vi "Analysis Info Cluster from String.vi"(7 "Setup String":string) -> (0 "Initial Probe Positions":T8[](array[typedef]), 1 "Dynamically Added":T1[](array[typedef]) {"Fs" format="%#_pHz"; "syncDelay" format="%#_gms"; "Ch" min=0 step=1}, 2 "XYZ Positions":dbl[][](array[numeric]), 3 "Ch & spans choices":T1[](array[typedef]) {"Fs" format="%#_pHz"; "syncDelay" format="%#_gms"; "Ch" min=0 step=1}, 4 "Initial Info Cluster":T7[](array[typedef]), 5 "Number of Analogue instruments":i32=1, 6 "Acquisition_Plugin":string[](array[string]), 8 "LDA Setup":T1[](array[typedef]) {"Fs" format="%#_pHz"; "syncDelay" format="%#_gms"; "Ch" min=0 step=1})   [LabVIEW 2022 SP3]
uses:
  Controls/Meas input Cluster.ctl
  Controls/Inst_type.ctl
  Controls/portOrDev.ctl
  Controls/calType.ctl
  Controls/channelState.ctl
  Controls/DAQinputType.ctl
  Controls/Initial Positions.ctl
  Controls/Initial Info Cluster.ctl
  Globals/Meas_global.vi
panel:
  in  "Inst type":T2=enum."Propeller anemometer"
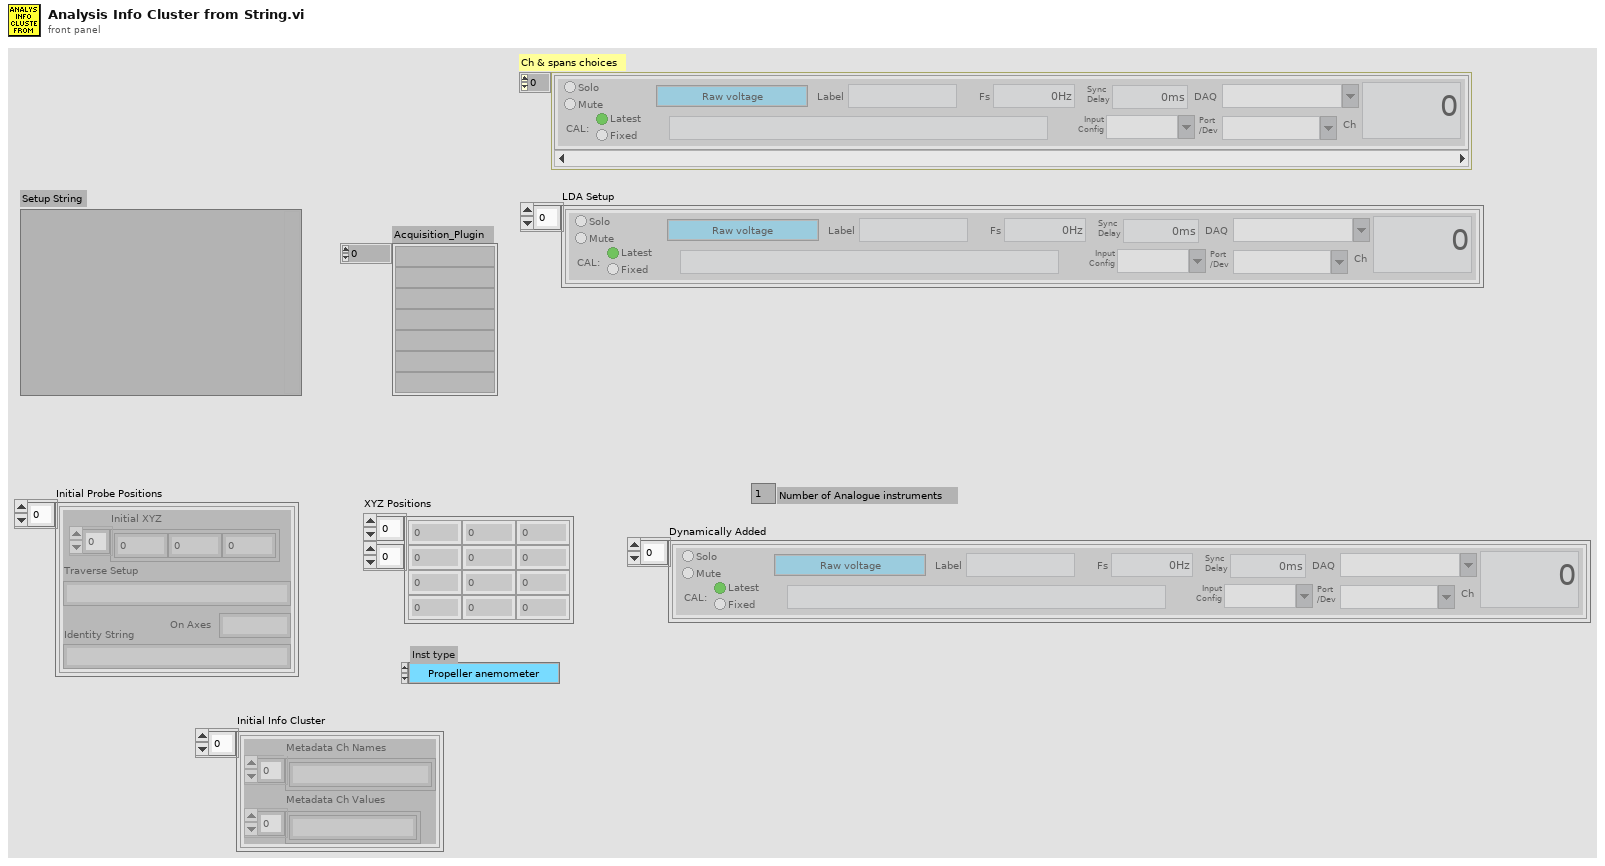
[diagram p1: front panel]
types:
  T1 = typedef "Meas input Cluster.ctl" = cluster{"Type":T2, "Label":string, "DAQ":string, "Port":T3, "Ch":i32, "Cal":path, "calType":T4, "Fs":dbl, "syncDelay":dbl, "chState":T5, "inputConfig":T6}
  T2 = typedef "Inst_type.ctl" = enum16{"Raw voltage", "Raw with zero offsetting", "Propeller anemometer", "Pressure Transducer", "Pitot-static tube", "Hot wire", "Cross wire 1", "Cross wire 2", "Generic Linear", "Generic Polynomial", "Generic BackPoly", "Fast FID", "Thermocouple", "Cold wire", "Pulsed Wire", "LDA Vel", "LDA Tran time", "LDA Arr time", "Microphone"}
  T3 = typedef "portOrDev.ctl" = string
  T4 = typedef "calType.ctl" = enum32{"Latest", "Fixed"}
  T5 = typedef "channelState.ctl" = enum32{"No Selection", "Solo", "Mute"}
  T6 = typedef "DAQinputType.ctl" = string
  T7 = typedef "Initial Info Cluster.ctl" = cluster{"Metadata Ch Names":string[], "Metadata Ch Values":string[]}
  T8 = typedef "Initial Positions.ctl" = cluster{"Initial XYZ":sgl[], "Traverse Setup":string, "On Axes":string, "Identity String":string}
  T9 = typedef "Post_Process.ctl" = enum16{"Take New Data", "Post Process Raw Data File"}
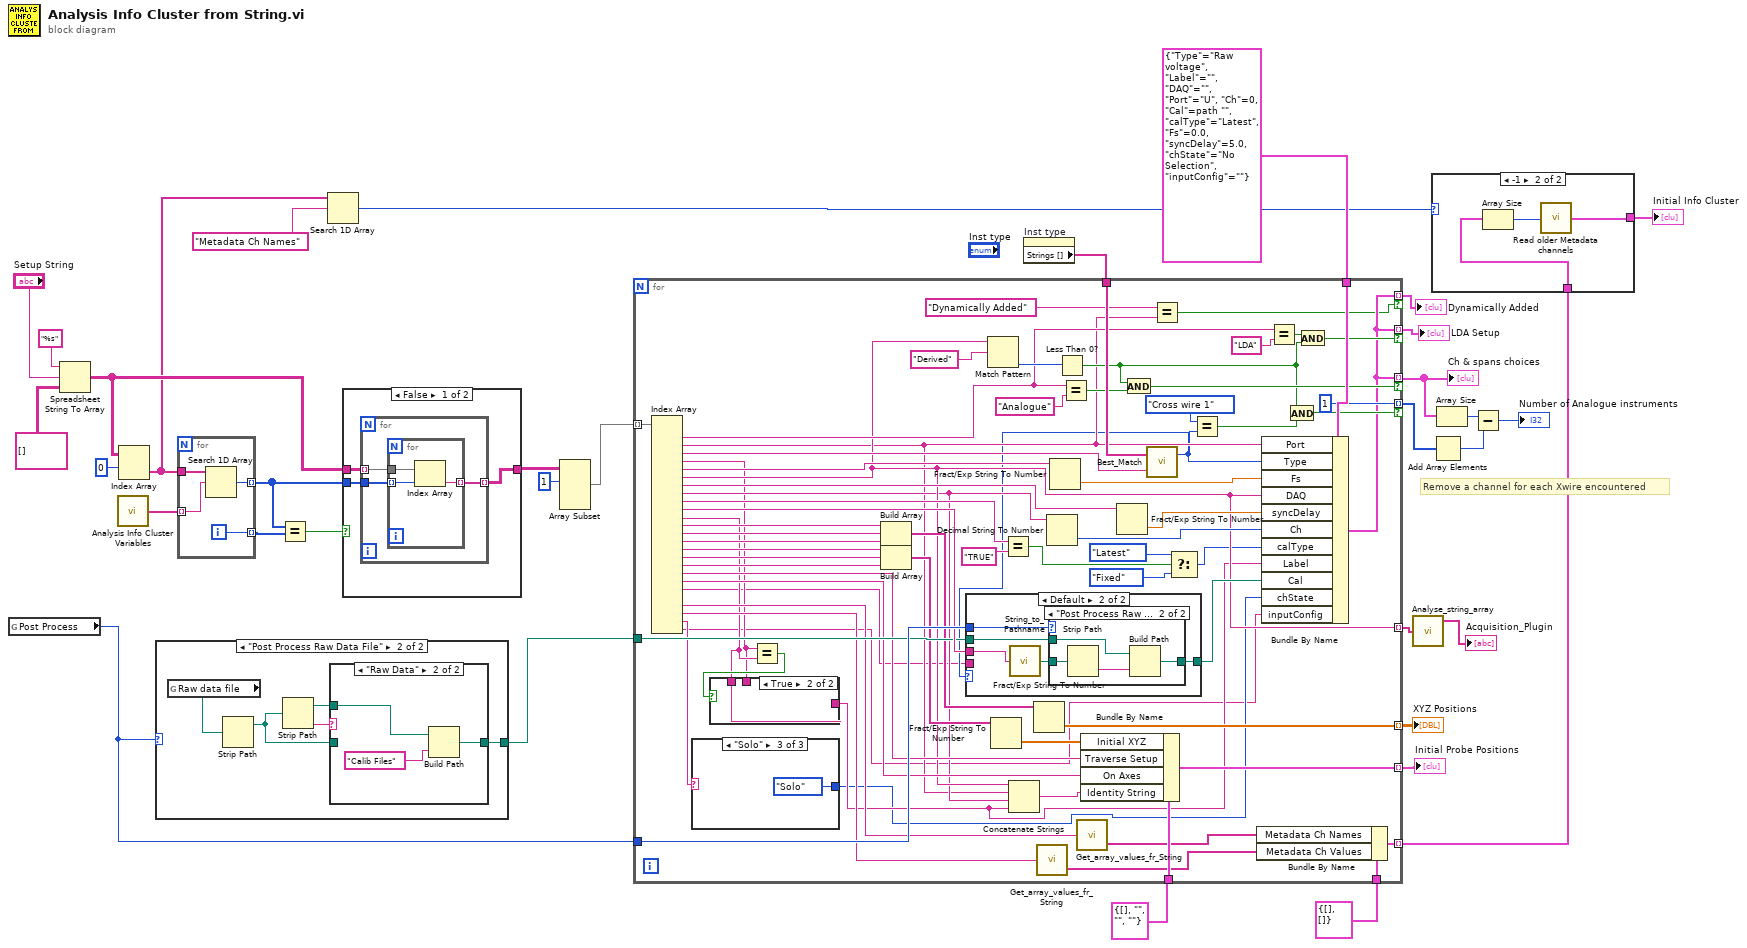
[diagram p0: block diagram]
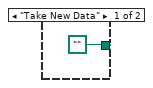
[diagram p4: hidden frame]
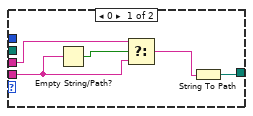
[diagram p6: hidden frame]
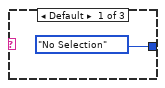
[diagram p8: hidden frame]
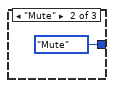
[diagram p9: hidden frame]
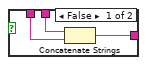
[diagram p10: hidden frame]
diagram:
  # "Remove a channel for each Xwire encountered"
  n1 = global read "Meas_global.vi" "Post Process"() -> (w30:T9)
  n2 = Spreadsheet String To Array(format string="%s", spreadsheet string="Setup String", array type (2D Dbl)=string[][] []) -> (array=w27:string[][])  [unwired: 1 in]
  n3 = call "Analysis Info Cluster Variables.vi"() -> ("Array"=w24:string[])
  n4 = Index Array(array=w27, index (row)=0) -> (element=w13:string[])  [unwired: 1 in]
  n5 = case shown="\"Post Process Raw Data File\"" w30 {
    tunnel: [path "" ("stripped path") w38] -> w29
    frame "Take New Data" {
    }
    frame "Post Process Raw Data File" {
      n6 = global read "Meas_global.vi" "Raw data file"() -> (w40:path)
      n7 = Strip Path(path=w40) -> (stripped path=w39:path)  [unwired: 1 out]
      n8 = Strip Path(path=w39) -> (stripped path=w36:path, name=w37:string)
      n9 = case shown="\"Raw Data\"" w37 {
        tunnel: w39 -> [w41 _]
        tunnel: [w41 w42] -> w38
        tunnel: w36 -> [_ w44]
        frame Default {
        }
        frame "Raw Data" {
          n10 = Build Path(base path=w44, name or relative path="Calib Files" ("format string")) -> (appended path=w42:path)
        }
      }
    }
  }
  n11 = for {
    tunnel: w13 -> [w48]
    tunnel: w24 -> [w47] mode=indexing
    tunnel: [w46] -> w23 mode=indexing
    tunnel: [w45] -> w22 mode=indexing
    i -> [w45]
    n12 = Search 1D Array(1D array=w48, element=w47) -> (index of element=w46:i32)  [unwired: 1 out]
  }
  n13 = Equal?(x=w23, y=w22) -> (x = y?=w21:bool)
  n14 = Search 1D Array(1D array=w13, element="Metadata Ch Names") -> (index of element=w11:i32)  [unwired: 1 out]
  n15 = case shown="False" w21 {
    tunnel: w27 -> [w51 w58]
    tunnel: [w50 w58] -> w26
    tunnel: w23 -> [w49 _]
    frame False {
      n16 = for {
        tunnel: w51 -> [w54] mode=indexing
        tunnel: w49 -> [w53]
        tunnel: [w52] -> w50 mode=indexing
        n17 = for {
          tunnel: w54 -> [w57]
          tunnel: w53 -> [w56] mode=indexing
          tunnel: [w55] -> w52 mode=indexing
          n18 = Index Array(array=w57, index=w56) -> (element=w55:string)
        }
      }
    }
    frame True {
    }
  }
  n19 = Array Subset(array=w26, index (row)=1 ("index")) -> (w28:string[][])  [unwired: 3 in]
  n20 = property on="Inst type" class="Enum (strict)"() -> ("Strings []"=w31:string[])  [unwired: 2 in, 2 out]
  n21 = for {
    tunnel: w28 -> [w127] mode=indexing
    tunnel: [w73] -> w15 mode=indexing if=w89
    tunnel: w31 -> [w126]
    tunnel: w30 -> [w118]
    tunnel: w29 -> [w116]
    tunnel: [w109] -> w20 mode=indexing
    tunnel: T8 {"Initial XYZ"=[], "Traverse Setup"="", "On Axes"="", "Identity String"=""} ("Initial Positions 3") -> [w105]
    tunnel: [w101] -> w17 mode=indexing
    tunnel: T1 {"Type"=enum."Raw voltage", "Label"="", "DAQ"="", "Port"="U", "Ch"=0, "Cal"=path "", "calType"=enum."Latest", "Fs"=0.0, "syncDelay"=5.0, "chState"=enum."No Selection", "inputConfig"=""} ("Cluster") -> [w99]
    tunnel: T7 {"Metadata Ch Names"=[], "Metadata Ch Values"=[]} ("Cluster") -> [w98]
    tunnel: [w97] -> w9 mode=indexing
    tunnel: [w78] -> w8 mode=indexing
    tunnel: [w73] -> w7 mode=indexing if=w85
    tunnel: [1] -> w4 mode=indexing if=w80
    tunnel: [w73] -> w1 mode=indexing if=w72
    n22 = Index Array(array=w127) -> (element #1=w87:string, element #2=w74:string, element #3=w125:string, element #4=w69:string, element #5=w124:string, element #6=w78:string, element #7=w122:string, element #8=w76:string, element #9=w120:string, element #10=w117:string, element #11=w70:string, element #12=w113:string, element #13=w112:string, element #14=w111:string, element #15=w108:string, element #16=w107:string, element #17=w106:string, element #18=w100:string, element #19=w102:string, element #20=w60:string, element #22=w96:string, element #23=w95:string, element #24=w63:string, element #25=w59:string)  [unwired: 25 in, 1 out]
    n23 = case shown="\"Solo\"" w63 {
      tunnel: [channelState."No Selection" ("chState") channelState."Mute" ("chState") channelState."Solo" ("chState")] -> w62
      frame Default {
      }
      frame "Mute" {
      }
      frame "Solo" {
      }
    }
    n24 = Equal?(x=w69, y=w70) -> (x = y?=w71:bool)
    n25 = case shown="True" w71 {
      tunnel: [w146 w149] -> w68
      tunnel: w70 -> [w147 w149]
      tunnel: w69 -> [w148 _]
      frame False {
        n26 = Concatenate Strings(w148, w147) -> (w146:string)
      }
      frame True {
      }
    }
    n27 = Build Array(w113, w112, w111) -> (w110:string[])
    n28 = Build Array(w108, w107, w106) -> (w104:string[])
    n29 = Match Pattern(string=w78, regular expression="Derived") -> (offset past match=w91:i32)  [unwired: 1 in, 3 out]
    n30 = Fract/Exp String To Number(string=w104) -> (number=w103:dbl[])  [unwired: 3 in, 1 out]
    n31 = Equal?(x=w120, y="TRUE") -> (x = y?=w67:bool)
    n32 = Concatenate Strings(w78, w74, w76, w68) -> (w77:string)
    n33 = Fract/Exp String To Number(string=w110) -> (number=w109:dbl[])  [unwired: 3 in, 1 out]
    n34 = call "Get_array_values_fr_String.vi"("String Value"=w95) -> ("String array"=w93:string[])  [unwired: 1 out]
    n35 = Decimal String To Number(string=w76) -> (number=w114:i32)  [unwired: 2 in, 1 out]
    n36 = Fract/Exp String To Number(string=w124) -> (number=w123:dbl)  [unwired: 3 in, 1 out]
    n37 = Less Than 0?(x=w91) -> (x < 0?=w79:bool)
    n38 = Equal?(x=w87, y="Analogue") -> (x = y?=w90:bool)
    n39 = call "Get_array_values_fr_String.vi"("String Value"=w96) -> ("String array"=w94:string[])  [unwired: 1 out]
    n40 = Bundle By Name(cluster=w105, "Initial XYZ"=w103, "Traverse Setup"=w100, "On Axes"=w102, "Identity String"=w77) -> (w101:T8)
    n41 = Fract/Exp String To Number(string=w122) -> (number=w121:dbl)  [unwired: 3 in, 1 out]
    n42 = And(x=w79, y=w90) -> (x .and. y?=w89:bool)
    n43 = call "Best_Match.vi"("Input String"=w125, "String Options"=w126) -> ("index of element"=w61:i32)  [unwired: 1 out]
    n44 = case shown="Default" w61 {
      tunnel: w118 -> [_ w137]
      tunnel: w117 -> [w130 w136]
      tunnel: w116 -> [_ w135]
      tunnel: [w132 w134] -> w84
      tunnel: w60 -> [w129 _]
      frame 0 {
        n45 = Empty String/Path?(string/path=w129) -> (empty?=w131:bool)
        n46 = Select(t=w130, s=w131, f=w129) -> (s? t:f=w128:string)
        n47 = String To Path(string=w128) -> (path=w132:path)
      }
      frame Default {
        n48 = call "String_to_Pathname.vi"("Input String"=w136) -> ("path"=w133:path)
        n49 = case shown="\"Post Process Raw Data File\"" w137 {
          tunnel: w133 -> [w138 w139]
          tunnel: [w138 w141] -> w134
          tunnel: w135 -> [_ w140]
          frame "Take New Data" {
          }
          frame "Post Process Raw Data File" {
            n50 = Strip Path(path=w139) -> (name=w142:string)  [unwired: 1 out]
            n51 = Build Path(base path=w140, name or relative path=w142) -> (appended path=w141:path)
          }
        }
      }
    }
    n52 = Equal?(x="Dynamically Added" ("Port"), y=w74) -> (x = y?=w72:bool)
    n53 = Select(t=calType."Latest" ("calType"), s=w67, f=calType."Fixed" ("calType")) -> (s? t:f=w64:T4)
    n54 = Equal?(x=Inst_type."Cross wire 1" ("Inst type"), y=w61) -> (x = y?=w81:bool)
    n55 = Bundle By Name(cluster=w98, "Metadata Ch Names"=w94, "Metadata Ch Values"=w93) -> (w97:T7)
    n56 = Bundle By Name(cluster=w99, "Port"=w74, "Type"=w61, "Fs"=w123, "DAQ"=w78, "syncDelay"=w121, "Ch"=w114, "calType"=w64, "Label"=w68, "Cal"=w84, "chState"=w62, "inputConfig"=w59) -> (w73:T1)
    n57 = Equal?(x=w87, y="LDA") -> (x = y?=w86:bool)
    n58 = And(x=w79, y=w81) -> (x .and. y?=w80:bool)
    n59 = And(x=w86, y=w79) -> (x .and. y?=w85:bool)
  }
  "Ch & spans choices" <- w15
  "XYZ Positions" <- w20
  "Initial Probe Positions" <- w17
  "LDA Setup" <- w7
  "Dynamically Added" <- w1
  n60 = call "Analyse_string_array.vi"("String array"=w8) -> ("Unique strings"=→"Acquisition_Plugin":string[])  [unwired: 1 in, 1 out]
  n61 = case shown="-1" w11 {
    tunnel: [w150 w153] -> w10
    tunnel: w9 -> [w150 w152]
    frame Default {
    }
    frame -1 {
      n62 = Array Size(array=w152) -> (size(s)=w151:i32)
      n63 = call "Read older Metadata channels.vi"("Number of Channels"=w151) -> ("Initial Info Cluster"=w153:T7[])
    }
  }
  "Initial Info Cluster" <- w10
  n64 = Add Array Elements(numeric array=w4) -> (sum=w2:i32)
  n65 = Array Size(array=w15) -> (size(s)=w6:i32)
  n66 = Subtract(x=w6, y=w2) -> (x-y=→"Number of Analogue instruments":i32)
